vi "zher2k - Hermitian Matrix Rank-2k Update (CDB).vi"(4 "beta":dbl=1.0, 6 "alpha":cdb=1.0+0.0i, 7 "operation":T2 items=["Direct", "Conjugated & Transposed", "Transposed"], 8 "matrix C type":T1=3 items=["Lower Triangular"=2, "Upper Triangular"=3], 9 "C":T3, 10 "B":T3, 11 "A":T3) -> (0 "error":i32, 3 "zher2k":T3)   [LabVIEW 2024, in "NI_AALBLAS.lvlib"]
doc: "<p>Calculates the rank<span class=\"U+8211\">-</span>2k update of the upper or lower triangular component of a Hermitian matrix.</p>"
uses:
  NI_AALBLAS.lvlib
  ComplexMatrix.ctl
  LV_Transpose.ctl
  LV_UpLo.ctl
  Fucntion.ctl
  Order.ctl
  BLAS3 Utility(CDB).vi
  NI_Matrix.lvlib
panel:
  # "zher2k=alpha*A*conjg(B')+conjg(alpha)*B*conjg(A')+beta*C / \nzher2k=alpha*conjg(A')*B+conjg(alpha)*conjg(B')*A+beta*C"
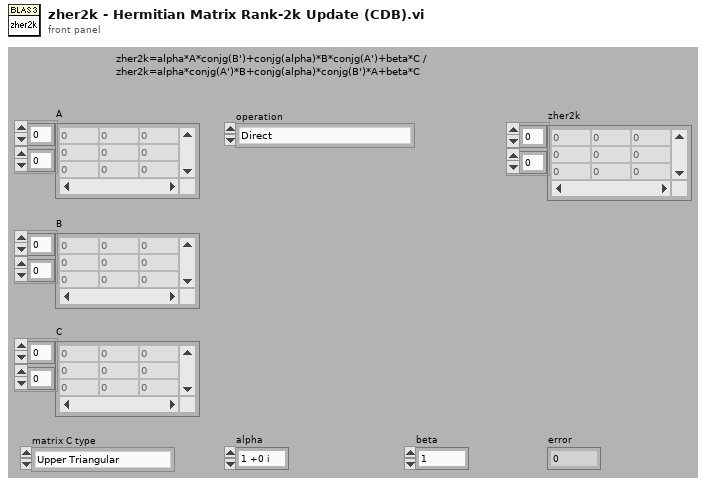
[diagram p1: front panel]
types:
  T1 = typedef "NI_AALBLAS.lvlib/LV_UpLo.ctl" = i32
  T2 = typedef "NI_AALBLAS.lvlib/LV_Transpose.ctl" = i32
  T3 = typedef "NI_Matrix.lvlib/ComplexMatrix.ctl" = cdb[][]
  T4 = typedef "NI_AALBLAS.lvlib/Order.ctl" = i32
  T5 = typedef "NI_AALBLAS.lvlib/Fucntion.ctl" = u16
  T6 = typedef "NI_AALBLAS.lvlib/UpLo.ctl" = i32
  T7 = typedef "NI_AALBLAS.lvlib/Operation_Transpose.ctl" = i32
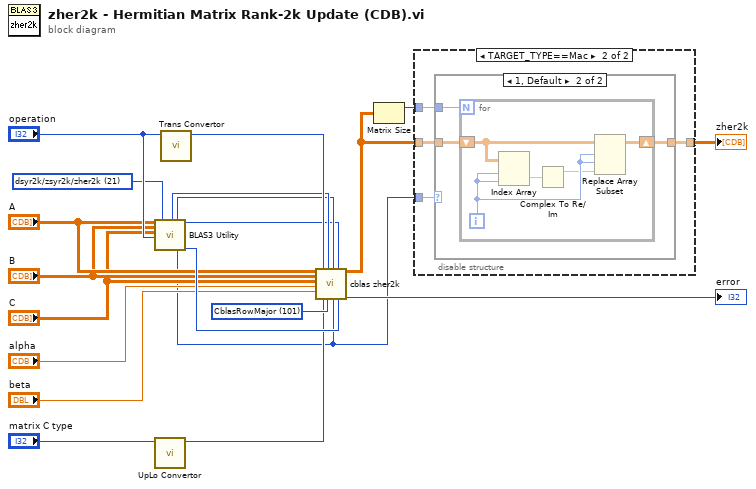
[diagram p0: block diagram]
diagram:
  w8 = T4 101 items=["CblasRowMajor"=101, "CblasColMajor"=102] ("order")
  w12 = T5 21 items=["ddot/zdotu/zdotc", "daxpy/zaxpy", "dnrm2/dznrm2", "dasum/dzasum", "dcopy/zcopy", "dswap/zswap", "drotm", "drot/zdrot", "idamax/izamax", "idamin/izamin", "dgemv/zgemv", "dsymv/zhemv", "dtrmv/ztrmv", "dsyr/zher", "dsyr2/zher2", "dger/zgeru/zgerc", "dtrsv/ztrsv", "dgemm/zgemm", "dsymm/zsymm/zhemm", "dtrmm/ztrmm", "dsyrk/zsyrk/zherk", "dsyr2k/zsyr2k/zher2k", "dtrsm/ztrsm"] ("function")
  n1 = call-poly "BLAS3 Utility.vi"("A"="A", "B/X"="B", "C"="C", "operation A"="operation", "function"=w12) -> ("lda"=w11:i32, "ldb/ldx"=w10:i32, "n"=w2:i32, "ldc"=w9:i32, "k"=w19:i32)  [unwired: 1 in, 9 out]
  n2 = call "UpLo Convertor.vi"("triangle matrix type"="matrix C type") -> ("uplo"=w6:T6)  [unwired: 10 out]
  n3 = call "Trans Convertor.vi"("operation"="operation") -> ("trans"=w15:T7)  [unwired: 10 out]
  n4 = call "cblas zher2k.vi"("A"="A", "B"="B", "C"="C", "alpha"="alpha", "beta"="beta", "order"=w8, "trans"=w15, "uplo"=w6, "lda"=w11, "ldb"=w10, "n"=w2, "ldc"=w9, "k"=w19) -> ("zher2k"=w4:T3, "error"=→"error":i32)  [unwired: 5 out]
  n5 = Matrix Size(0:w4) -> (1:w1:i32)  [unwired: 1 out]
  n6 = disable-structure shown="TARGET_TYPE==Mac" {
    disable-tunnel: w4 -> [w21 w25]
    disable-tunnel: [w21 w24] -> w3
    disable-tunnel: w2 -> [_ w23]
    disable-tunnel: w1 -> [_ w22]
    frame condition #0 (active) {
    }
    frame condition #1 {
      n7 = case shown="1, Default" w23 {
        tunnel: w25 -> [w26 w29]
        tunnel: [w26 w28] -> w24
        tunnel: w22 -> [_ w27]
        frame 0 {
        }
        frame 1, Default {
          n8 = for {
            N: w27 -> [_]
            shift-right: [w34] -> w28
            shift-left: w29 -> [w33]
            i -> [w31]
            n9 = Index Array(array=w33, index (row)=w31, index (col)=w31) -> (element=w32:cdb)
            n10 = Complex To Re/Im(x + iy=w32) -> (x=w30:dbl)  [unwired: 1 out]
            n11 = Replace Array Subset(array=w33, new element=w30, index (row)=w31, index (col)=w31) -> (w34:T3)
          }
        }
      }
    }
  }
  "zher2k" <- w3
